vi "132CAM1CAM2.vi"() -> ()   [LabVIEW 2019]
panel:
  out "Boolean":bool
  in  "CAM3":bool=TRUE
  in  "CAM4":bool=TRUE
  in  "error in":errorcluster
  out "error out":errorcluster
  out "APX HPC BOTTOM OV":T1(plugin-control)
  out "APX HPC BOTTOM APERTURE":T1(plugin-control)
  out "APX HPC SIDE EDGE":T1(plugin-control)
  out "APX HPC SIDE CONE":T1(plugin-control)
  out "APX HPC SIDE OV":T1(plugin-control)
  in  "stop":bool
  # "26u/pixel"
  # "0.5mm"
  # "12mm"
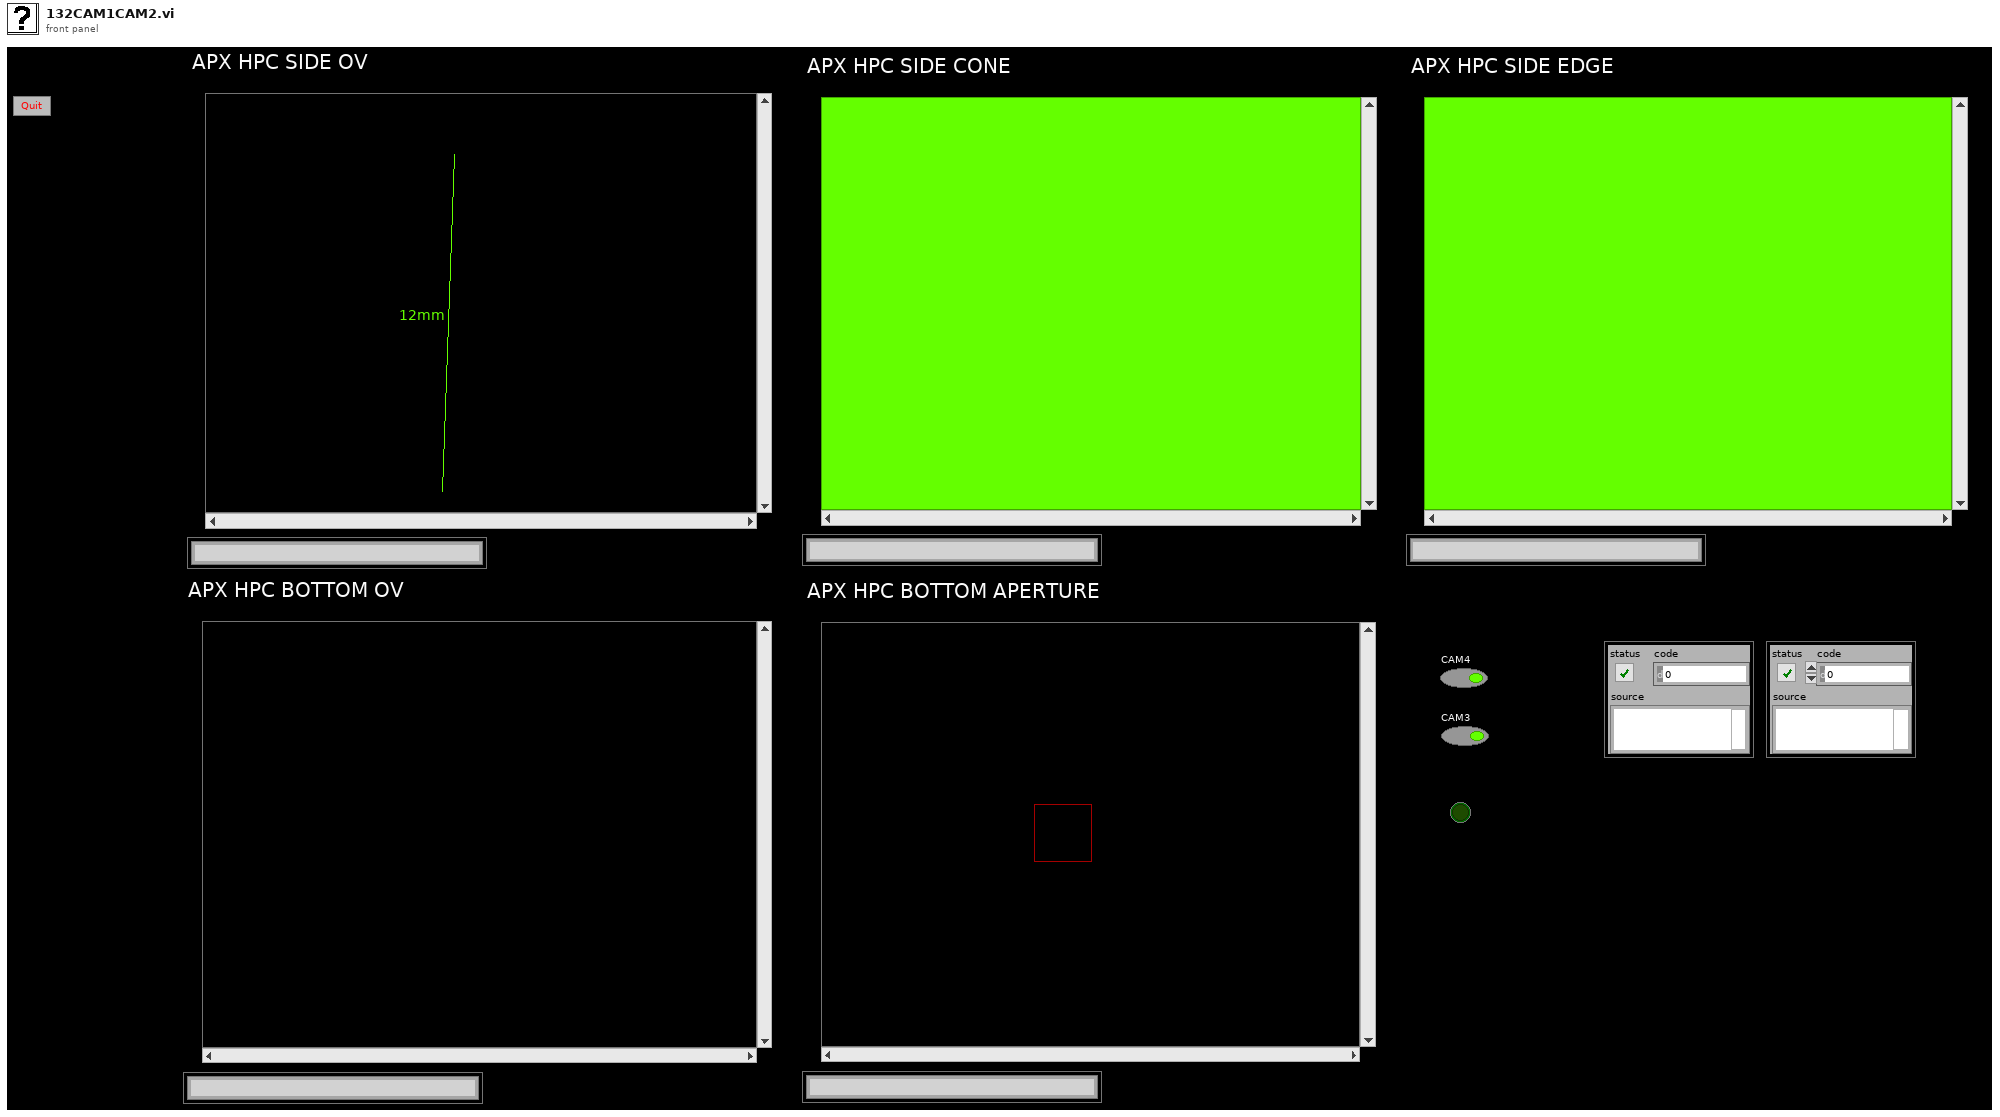
[diagram p1: front panel]
types:
  T1 = typedef "IMAQ Image.ctl" = refnum<image>
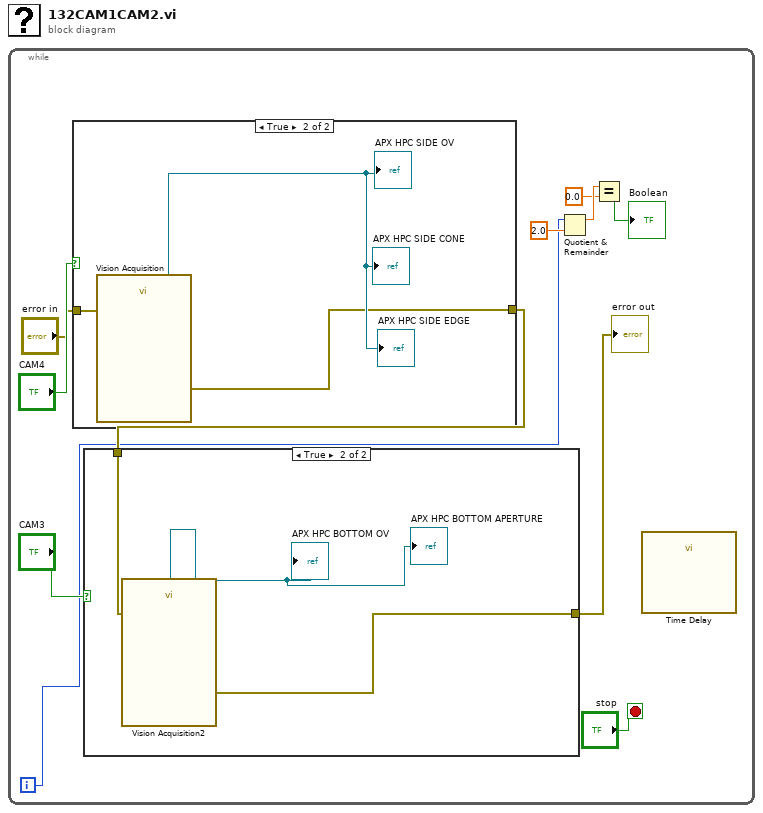
[diagram p0: block diagram]
diagram:
  n1 = while {
    i -> [w2]
    stop <- "stop" stop-if-true
    n2 = case shown="True" "CAM4" {
      tunnel: [w16 w18] -> w7
      tunnel: "error in" -> [w16 w17]
      frame False {
      }
      frame True {
        n3 = call "Vision Acquisition"("error in"=w17) -> ("Image Out"=→"APX HPC SIDE OV" →"APX HPC SIDE CONE" →"APX HPC SIDE EDGE":T1, "error out"=w18:errorcluster)  [unwired: 24 in, 1 out]
      }
    }
    n4 = case shown="True" "CAM3" {
      tunnel: w7 -> [w12 w14]
      tunnel: [w12 w13] -> w6
      frame False {
      }
      frame True {
        n5 = call "Vision Acquisition2"("error in"=w14) -> ("Image Out"=→"APX HPC BOTTOM OV" →"APX HPC BOTTOM APERTURE":T1, "error out"=w13:errorcluster)  [unwired: 24 in, 1 out]
      }
    }
    "error out" <- w6
    n6 = Quotient & Remainder(x=w2, y=2.0) -> (x-y*floor(x/y)=w5:dbl)  [unwired: 1 out]
    n7 = Equal?(x=w5, y=0.0) -> (x = y?=→"Boolean":bool)
    n8 = call "Time Delay"() -> ()  [unwired: 11 in, 1 out]
  }
